vi "Unpack Auto Step.vi"(11 "Step Array":dbl[](array[numeric])) -> (0 "Arg3":dbl, 1 "Arg2":dbl, 2 "Arg1":dbl, 3 "Args":dbl[](array[numeric]), 4 "Arg4":dbl, 5 "Step Type":T1, 6 "Timeout":u32)   [LabVIEW 2017]
uses:
  Auto Actions.ctl
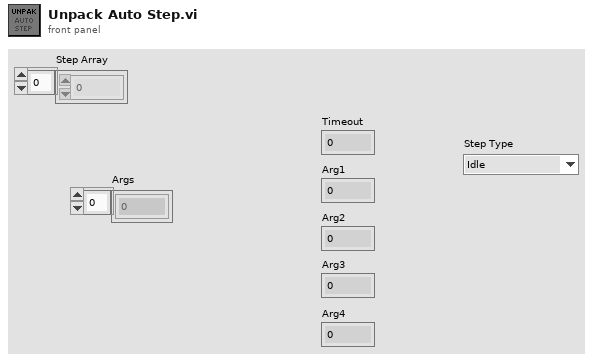
[diagram p1: front panel]
types:
  T1 = typedef "Auto Actions.ctl" = enum16{"Idle", "Drive", "Turn", "Lift", "Cube"}
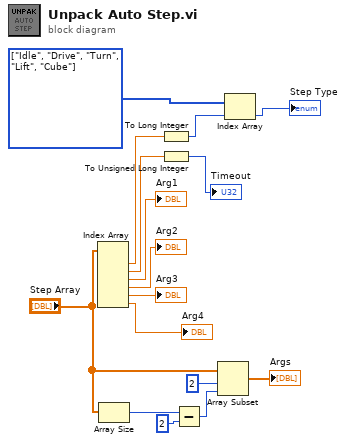
[diagram p0: block diagram]
diagram:
  w3 = T1[] [enum."Idle", enum."Drive", enum."Turn", enum."Lift", enum."Cube"] items=["Idle", "Drive", "Turn", "Lift", "Cube"] ("Array")
  n1 = Index Array(array="Step Array") -> (element #1=w8:dbl, element #2=w7:dbl, element #3=→"Arg1":dbl, element #4=→"Arg2":dbl, element #5=→"Arg3":dbl, element #6=→"Arg4":dbl)  [unwired: 6 in]
  n2 = Array Size(array="Step Array") -> (size(s)=w9:i32)
  n3 = To Long Integer(number=w8) -> (32bit integer=w2:i32)
  n4 = To Unsigned Long Integer(number=w7) -> (unsigned 32bit integer=→"Timeout":u32)
  n5 = Subtract(x=w9, y=2) -> (x-y=w10:i32)
  n6 = Array Subset(array="Step Array", index=2, length=w10) -> (→"Args":dbl[])
  n7 = Index Array(array=w3, index=w2) -> (element=→"Step Type":T1)
